vi "Comm_open 2d cdb waveform.vi"(6 "Access":T2, 7 "Communication Properties":T1={"WPL"={"Custom Queue Size"=1, "Use Custom Queue Size?"=FALSE}}, 8 "error in (no error)":errorcluster, 9 "dt":dbl=nan, 10 "Waveform Data References":i32[](array[numeric]), 11 "WPL Comm (2D CDB) in":refnum<class "WPL Comm (2D CDB).lvclass">) -> (0 "error out":errorcluster, 3 "WPL Comm (2D CDB) out":refnum<class "WPL Comm (2D CDB).lvclass">)   [LabVIEW 2020, in "Internal Comm Classes.lvlib" / "WPL Comm (2D CDB).lvclass"]
uses:
  WPL Comm (2D CDB).lvclass
  D:/p4/penguin/lvaddon/Veristand/master/src/LabVIEW/vilib/NI VeriStand/Custom Device Waveform API/Internal Comm Classes/WPL Comm/WPL Comm.lvclass
  Access mode.ctl
  Communication Properties.ctl
  WPL Comm (2D CDB).lvclass/WPL Comm (2D CDB).ctl
  WPL Command.ctl
  WPL Comm.lvclass/WPL Comm.ctl
  Send WPL Command.vi
  Set ErrorQ on Variant.vi
  Set dt on Variant.vi
  Error Check Empty Ref Array.vi
  Convert Q Error to Shutdown Error.vi
  WPL Comm.lvclass
  NI_VS Custom Device Waveform API.lvlib
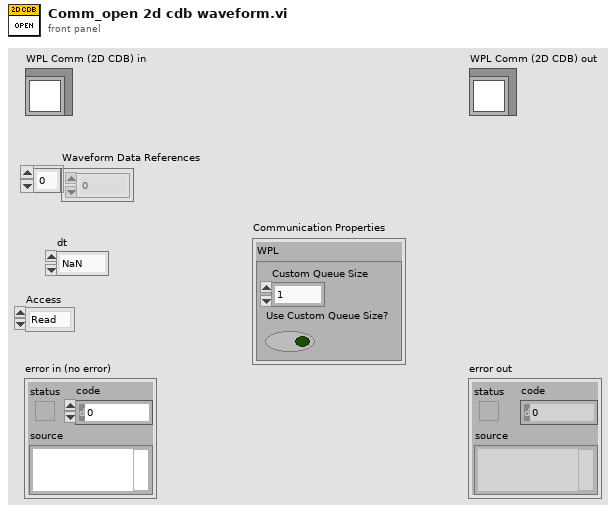
[diagram p1: front panel]
types:
  T1 = typedef "NI_VS Custom Device Waveform API.lvlib/Communication Properties.ctl" = cluster{"WPL":cluster{"Custom Queue Size":i32, "Use Custom Queue Size?":bool}}
  T2 = typedef "NI_VS Custom Device Waveform API.lvlib/Access mode.ctl" = enum16{"Read", "Write"}
  T3 = typedef "Internal Comm Classes.lvlib/WPL Comm.lvclass/WPL Command.ctl" = enum16{"Register 1D DBL Reader", "Unregister 1D DBL Reader", "Register 1D DBL Writer", "Register 2D DBL Writer", "Unregister 1D DBL Writer", "Unregister 2D DBL Writer", "DBL WFM Start", "WFM 1D DBL Data", "WFM 2D DBL Data", "Shut down", "Handle Error", "Register 1D CDB Reader", "Unregister 1D CDB Reader", "Register 1D CDB Writer", "Unregister 1D CDB Writer", "Register 2D CDB Writer", "Unregister 2D CDB Writer", "WFM 1D CDB Data", "WFM 2D CDB Data", "CDB WFM Start", "Error Shutdown", "Register Streams", "Unregister Streams", "Delete All Streams", "Get WFM DTs", "DBL WFM Multi Start", "CDB WFM Multi Start"}
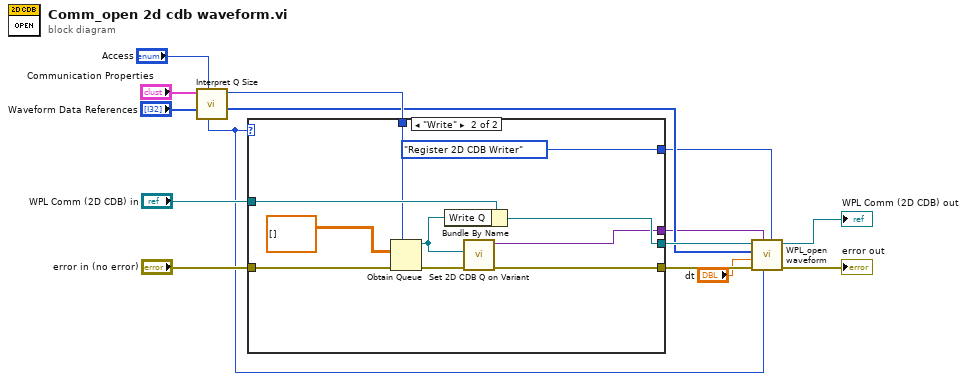
[diagram p0: block diagram]
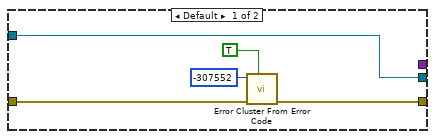
[diagram p2: hidden frame]
diagram:
  n1 = call "Interpret Q Size.vi"("Access"="Access", "Waveform Data References"="Waveform Data References", "Communication Properties"="Communication Properties") -> ("Waveform Data References dup"=w3:i32[], "Queue Size"=w7:i32, "Access dup"=w5:T2)  [unwired: 6 in]
  n2 = case shown="\"Write\"" w5 {
    tunnel: [w19 w25] -> w11
    tunnel: [w18 w23] -> w12
    tunnel: "error in (no error)" -> [w20 w30]
    tunnel: "WPL Comm (2D CDB) in" -> [w18 w28]
    tunnel: w7 -> [_ w27]
    tunnel: [_ WPL_Command."Register 2D CDB Writer" ("Command")] -> w2
    tunnel: [_ w21] -> w1
    frame Default {
      n3 = call <vilib>:"Error Cluster From Error Code.vi"("show call chain? (False)"=TRUE, "error in (no error)"=w20, "error code (0)"=-307552) -> ("error out"=w19:errorcluster)  [unwired: 6 in]
    }
    frame "Write" {
      n4 = Obtain Queue(max queue size (-1, unlimited)=w27, element data type=cdb[][] [], error in (no error)=w30) -> (queue out=w24:refnum<queue>, error out=w26:errorcluster)  [unwired: 2 in, 1 out]
      n5 = Bundle By Name(cluster=w28, "Write Q"=w24) -> (w23:refnum<class "WPL Comm (2D CDB).lvclass">)
      n6 = call "Set 2D CDB Q on Variant.vi"("error in (no error)"=w26, "2D CDB Data Q"=w24) -> ("error out"=w25:errorcluster, "Variant out"=w21:variant)  [unwired: 7 in, 1 out]
    }
  }
  n7 = call "WPL_open waveform.vi"("Command"=w2, "Access"=w5, "Variant in"=w1, "error in (no error)"=w11, "dt"="dt", "WFM Data Idx"=w3, "WPL Comm in"=w12) -> ("error out"=→"error out":errorcluster, "WPL Comm out"=→"WPL Comm (2D CDB) out":refnum<class "WPL Comm (2D CDB).lvclass">)  [unwired: 3 in]
